vi "Create DQMH Overview.vi"(8 "error in":errorcluster, 10 "DQMH Modules":refnum<class "Dqmh Module.lvclass">[](array[class])) -> (0 "error out":errorcluster, 3 "Dqmh Modules Overview out":refnum<class "Dqmh Modules Overview.lvclass">)   [LabVIEW 2021, in "TAF Proj Document Type.lvlib" / "Dqmh Modules Overview.lvclass"]
uses:
  <vilib>/Wovalab/AntiDoc/Document Type/Add-ons/LabVIEW TAF Project/Dqmh Modules Overview/Dqmh Modules Overview.lvclass
  C:/Program Files (x86)/National Instruments/LabVIEW 2021/vi.lib/Wovalab/AntiDoc/Bloc/Bloc.lvclass
  <vilib>/Wovalab/AntiDoc/Document Type/Add-ons/LabVIEW TAF Project/Dqmh Module/Dqmh Module.lvclass
  <vilib>/Wovalab/AntiDoc/Document Type/Add-ons/LabVIEW TAF Project/Dqmh Modules Overview/Dqmh Modules Overview.lvclass/Dqmh Modules Overview.ctl
  <vilib>/Wovalab/AntiDoc/Bloc/Bloc.lvclass/Bloc.ctl
  <vilib>/Wovalab/AntiDoc/Document Type/Add-ons/LabVIEW TAF Project/Dqmh Modules Overview/Write DQMH Modules.vi
  <vilib>/Wovalab/AntiDoc/Bloc/Write Name.vi
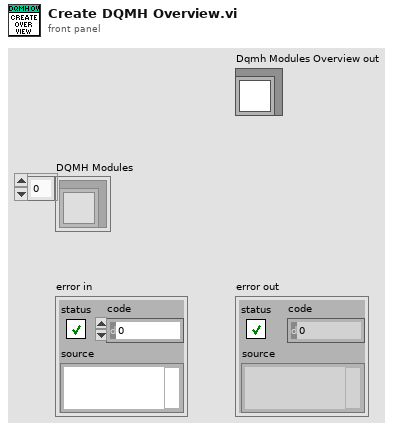
[diagram p1: front panel]
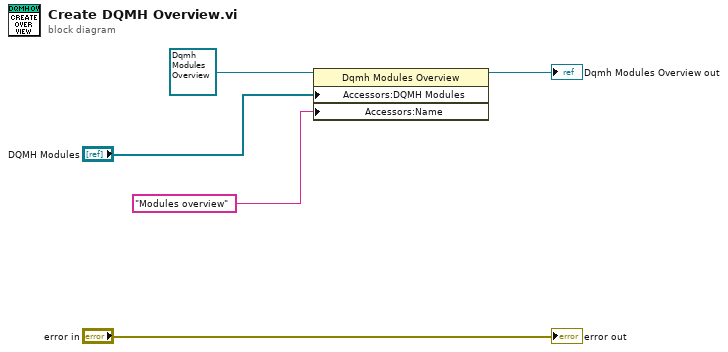
[diagram p0: block diagram]
diagram:
  n1 = property class="Dqmh Modules Overview"(reference=refnum<class "Dqmh Modules Overview.lvclass"> refnum ("Dqmh Modules Overview in"), "Accessors:DQMH Modules"="DQMH Modules", "Accessors:Name"="Modules overview" ("Title")) -> (reference out=→"Dqmh Modules Overview out":refnum<class "Dqmh Modules Overview.lvclass">)  [unwired: 1 in, 1 out]
  "error out" <- "error in"
